vi "Griper_Control_PID.vi"() -> ()   [LabVIEW 2019]
uses:
  <vilib>/addons/control/pid/NI_PID_pid.lvlib
  <vilib>/addons/control/pid/pid.llb/PID (DBL).vi
panel:
  out "Posicion (°)":cluster{dbl, "SetPoint":dbl}(graph)
  in  "Rangos de Salida":cluster{"output high":dbl, "output low":dbl}
  in  "Gain PID":T1 {"derivative time (Td, min)" scale=0.0..10.0; "integral time (Ti, min)" scale=0.0..10.0; "proportional gain (Kc)" scale=0.0..10.0}
  in  "Reinicializar":bool
  out "dt out (s)":dbl
  in  "dt (s)":dbl
  in  "SetPoint":dbl(slide) scale=-360.0..360.0
  out "Sensor_5 2":dbl
  out "Sensor_4 2":dbl
  in  "Señal_5 2":dbl
  in  "Señal_4 2":dbl
  in  "Señal_3 2":dbl
  in  "Señal_2 2":dbl
  in  "Señal_1 2":dbl
  out "Trama de envio 2":string
  out "Sensor_3 TOF":dbl
  out "Sensor_2 US2":dbl
  out "Sensor_1 US1":dbl
  out "Trama Recibida 2":string
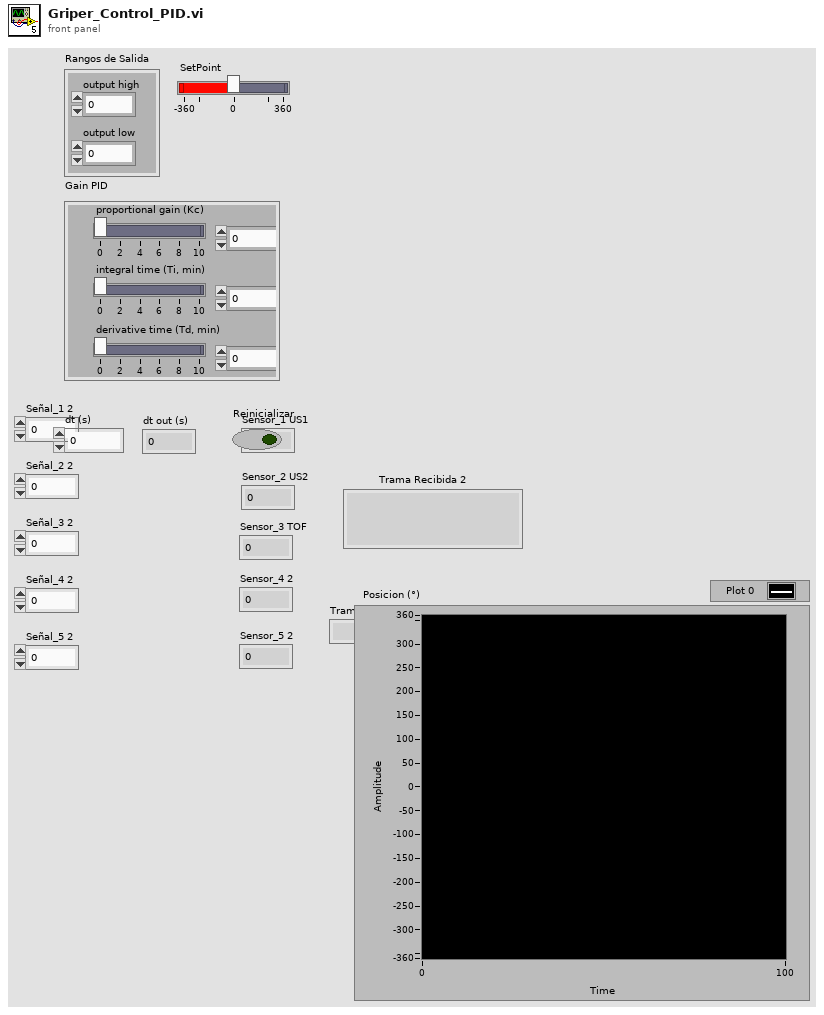
[diagram p1: front panel]
types:
  T1 = cluster{"proportional gain (Kc)":dbl, "integral time (Ti, min)":dbl, "derivative time (Td, min)":dbl}
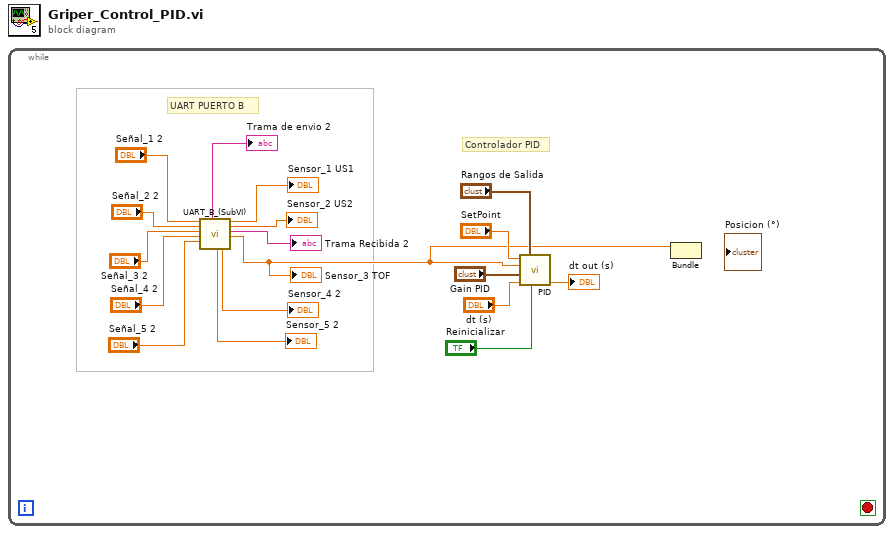
[diagram p0: block diagram]
diagram:
  n1 = while {
    stop <- _ stop-if-true
    # "Controlador PID"
    # "UART PUERTO B"
    n2 = call "UART_B_(SubVI).vi"("Señal_1 in"="Señal_1 2", "Señal_2 in"="Señal_2 2", "Señal_3 in"="Señal_3 2", "Señal 6"="Señal_4 2", "Señal 7"="Señal_5 2") -> ("Trama de envio 2"=→"Trama de envio 2":string, "Sensor 7"=→"Sensor_5 2":dbl, "Sensor 6"=→"Sensor_4 2":dbl, "Sensor_1 2"=→"Sensor_1 US1":dbl, "Sensor_2 2"=→"Sensor_2 US2":dbl, "Trama Recibida 2"=→"Trama Recibida 2":string, "Sensor_3 2"=w1:dbl)  [unwired: 3 in, 5 out]
    "Sensor_3 TOF" <- w1
    n3 = call-poly <vilib>:"PID.vi"("reinitialize? (F)"="Reinicializar", "output range"="Rangos de Salida", "dt (s)"="dt (s)", "PID gains"="Gain PID", "process variable"=w1, "setpoint"="SetPoint") -> ("dt out (s)"=→"dt out (s)":dbl)  [unwired: 4 in, 1 out]
    n4 = Bundle("Sensor_3 2"=w1) -> ()  [unwired: 2 in, 1 out]
  }
